vi "getResponse.vi"(8 "error in (no error)":errorcluster, 9 "ST":u32, 10 "string":string, 11 "Bytes at Serial Port":u32) -> (0 "error out":errorcluster, 2 "responce":string, 3 "done":bool)   [LabVIEW 2022 SP3]
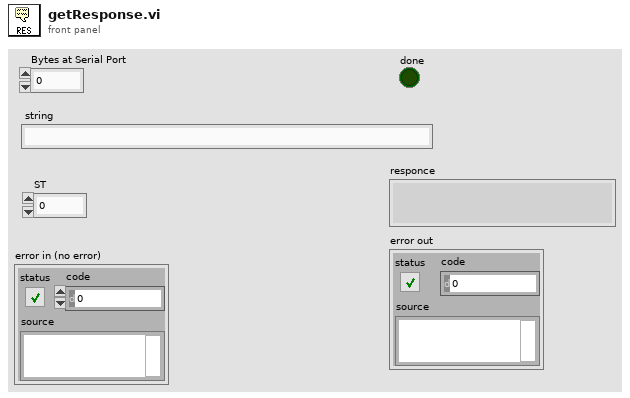
[diagram p1: front panel]
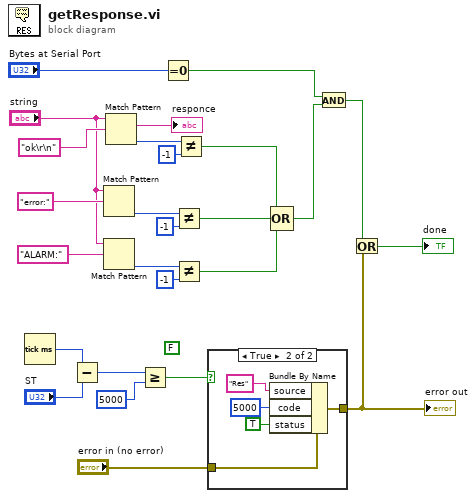
[diagram p0: block diagram]
diagram:
  (unwired) FALSE
  n1 = Tick Count (ms)() -> (millisecond timer value=w19:u32)
  n2 = Subtract(x=w19, y="ST") -> (x-y=w17:u32)
  n3 = Match Pattern(string="string", regular expression="error:" ("response")) -> (offset past match=w9:i32)  [unwired: 1 in, 3 out]
  n4 = Match Pattern(string="string", regular expression="ALARM:" ("response")) -> (offset past match=w5:i32)  [unwired: 1 in, 3 out]
  n5 = Match Pattern(string="string", regular expression="ok\r\n" ("response")) -> (match substring=→"responce":string, offset past match=w26:i32)  [unwired: 1 in, 2 out]
  n6 = Greater Or Equal?(x=w17, y=u32 5000) -> (x >= y?=w12:bool)
  n7 = Equal To 0?(x="Bytes at Serial Port") -> (x = 0?=w24:bool)
  n8 = Not Equal?(x=w9, y=-1) -> (x != y?=w7:bool)
  n9 = Not Equal?(x=w5, y=-1) -> (x != y?=w1:bool)
  n10 = Not Equal?(x=w26, y=-1) -> (x != y?=w8:bool)
  n11 = case shown="True" w12 {
    tunnel: "error in (no error)" -> [w27 w32]
    tunnel: [w27 w31] -> w14
    frame False {
    }
    frame True {
      n12 = Bundle By Name(cluster=w32, "source"="Res", "code"=5000, "status"=TRUE) -> (w31:errorcluster)
    }
  }
  "error out" <- w14
  n13 = Compound Arithmetic op=OR(w8, w7, w1) -> (w6:bool)
  n14 = And(x=w24, y=w6) -> (x .and. y?=w22:bool)
  n15 = Or(x=w22, y=w14) -> (x .or. y?=→"done":bool)
